vi "Bury.vi"(8 "Error In":errorcluster) -> (0 "Error Out":errorcluster)   [LabVIEW 2017, in "Tests.lvlib"]
uses:
  Tests.lvlib
  src/Toolkit VIs/Toolkit.lvlib
  <vilib>/addons/_JKI Toolkits/Caraya/classes/Test/Test.lvclass
  <vilib>/addons/_JKI Toolkits/Caraya/classes/Assert/Assert.lvclass
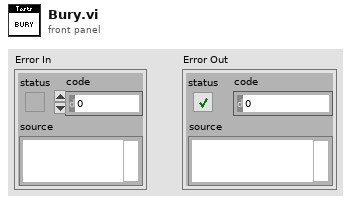
[diagram p1: front panel]
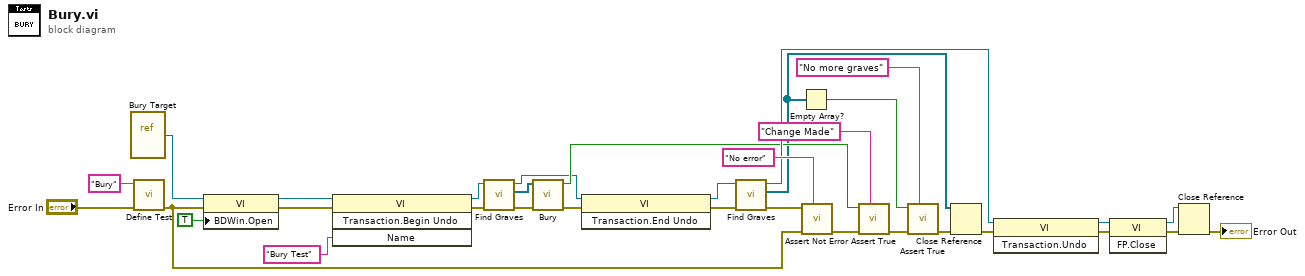
[diagram p0: block diagram]
diagram:
  n1 = vi-ref "Bury Target.vi"() -> (w1:refnum<vi>)
  n2 = call <vilib>:"Define Test.vi"("error in (no error)"="Error In", "Label (VI Title)"="Bury") -> ("error out"=w7:errorcluster)  [unwired: 9 in]
  n3 = property class="VI"(reference=w1, error in=w7, "BDWin.Open"=TRUE ("Block Diagram Window:Open")) -> (reference out=w8:refnum<vi>, error out=w6:errorcluster)
  n4 = invoke class="VI" method="Transaction.Begin Undo"(reference=w8, error in=w6, "Name"="Bury Test") -> (reference out=w14:refnum<vi>, error out=w16:errorcluster)  [unwired: 1 in, 2 out]
  n5 = call "Find Graves.vi"("Error In"=w16, "VI In"=w14) -> ("Error Out"=w15:errorcluster, "Graves"=w12:refnum<vi>[], "VI Out"=w13:refnum<vi>)  [unwired: 7 in]
  n6 = call "Bury.vi"("Error In"=w15, "Graves"=w12) -> ("Error Out"=w32:errorcluster, "Change Made?"=w18:bool)  [unwired: 8 in]
  n7 = invoke class="VI" method="Transaction.End Undo"(reference=w13, error in=w32) -> (reference out=w30:refnum<vi>, error out=w31:errorcluster)  [unwired: 1 in, 1 out]
  n8 = call "Find Graves.vi"("Error In"=w31, "VI In"=w30) -> ("Error Out"=w25:errorcluster, "Graves"=w9:refnum<vi>[], "VI Out"=w22:refnum<vi>)  [unwired: 7 in]
  n9 = Empty Array?(array=w9) -> (empty?=w11:bool)
  n10 = call <vilib>:"Assert Not Error.vi"("Label"="No error", "error in (no error)"=w7, "Not Error?"=w25) -> ("error out"=w27:errorcluster)  [unwired: 8 in]
  n11 = call <vilib>:"Assert True.vi"("Label"="Change Made", "error in (no error)"=w27, "True?"=w18) -> ("error out"=w19:errorcluster)  [unwired: 8 in]
  n12 = call <vilib>:"Assert True.vi"("Label"="No more graves", "error in (no error)"=w19, "True?"=w11) -> ("error out"=w23:errorcluster)  [unwired: 8 in]
  n13 = Close Reference(reference=w9, error in (no error)=w23) -> (error out=w10:errorcluster)
  n14 = invoke class="VI" method="Transaction.Undo"(reference=w22, error in=w10) -> (reference out=w21:refnum<vi>, error out=w3:errorcluster)  [unwired: 1 in, 1 out]
  n15 = invoke class="VI" method="FP.Close"(reference=w21, error in=w3) -> (reference out=w4:refnum<vi>, error out=w2:errorcluster)  [unwired: 1 in, 1 out]
  n16 = Close Reference(reference=w4, error in (no error)=w2) -> (error out=→"Error Out":errorcluster)
